vi "BeEST Temperature Logger V4 (BASVR).vi"() -> ()   [LabVIEW 2023]
uses:
  <vilib>/Utility/miscctls.llb/LVRowAndColumnTypeDef.ctl
  <vilib>/Utility/Data Type/NI_Data Type.lvlib
panel:
  out "Expected Issue":string
  in  "Tab Control":enum32{"Setup", "Run", "Advanced"}(tab)
  in  "Calibration File Path":path=path "C:/Users/CK014-user/Desktop/AVS Code V4.2/BeEST Calibration Sheet.csv"
  in  "Logging File Path":path=path "C:/Users/CK014-user/Desktop/AVS Code V4.2/BeEST Temperature Logger V4 (BASVR)/Logs/Log1.tdms"
  in  "Record Group":string="10/1/2025"
  in  "VISA RESOURCE":refnum<visa-resource-name>="COM20"
  in  "Graph Samples":T1={"Start"="0", "Max Samples"=2500000, "End"="m"} {"Max Samples" min=1}
  out "Last Y Values":i32(listbox)=3
  in  "Elapsed":bool
  in  "Graph":bool=TRUE
  in  "Record":bool=TRUE
  in  "Graph Inputs":T2={"Group"="Measured Data", "Time Track"="TIME", "Value Track"="RESISTANCE (OHMS)", "Channel Track"="CHANNEL", "Range Track"="RANGE"}
  out "Recorded\nChannels":i32(listbox)
  in  "Channel Control & Legend":i32(listbox)=2
  out "Measuring (Channel)":i32
  in  "Measure Now":u16(ring) items=["None", "0", "1", "2", "3", "4", "5", "6", "7"]
  in  "Res. to Temp.":bool=TRUE
  in  "Moving Median":u8=30 min=1
  in  "Label Precision":i32=3
  in  "Override":bool
  in  "Override Controls":T3
  in  "Generate Random AVS Data":bool
  out "Started Measuring":timestamp
  out "Resistance (Ohms)":dbl
  out "Error Code":errorcluster
  out "EXCITATION":u8
  out "Chosen Channel Index":i32
  out "XY Graph":cluster{timestamp[], "Y Array":dbl[]}[](graph)
  # "• Moving median allows you to opt for noisier, and initially more misleading, data in exchange for earlier graphing of new data if you set it especially low.\n• Graphs can fail to read if range of data is just too wide (e.g. days, at least).  This is a common, virtually inevitable bug.\n• Supposed system errors are often user errors.  Always check what calibration file you're using, what names you're using in the legend, what group you're recording, what group you're reading, etc"
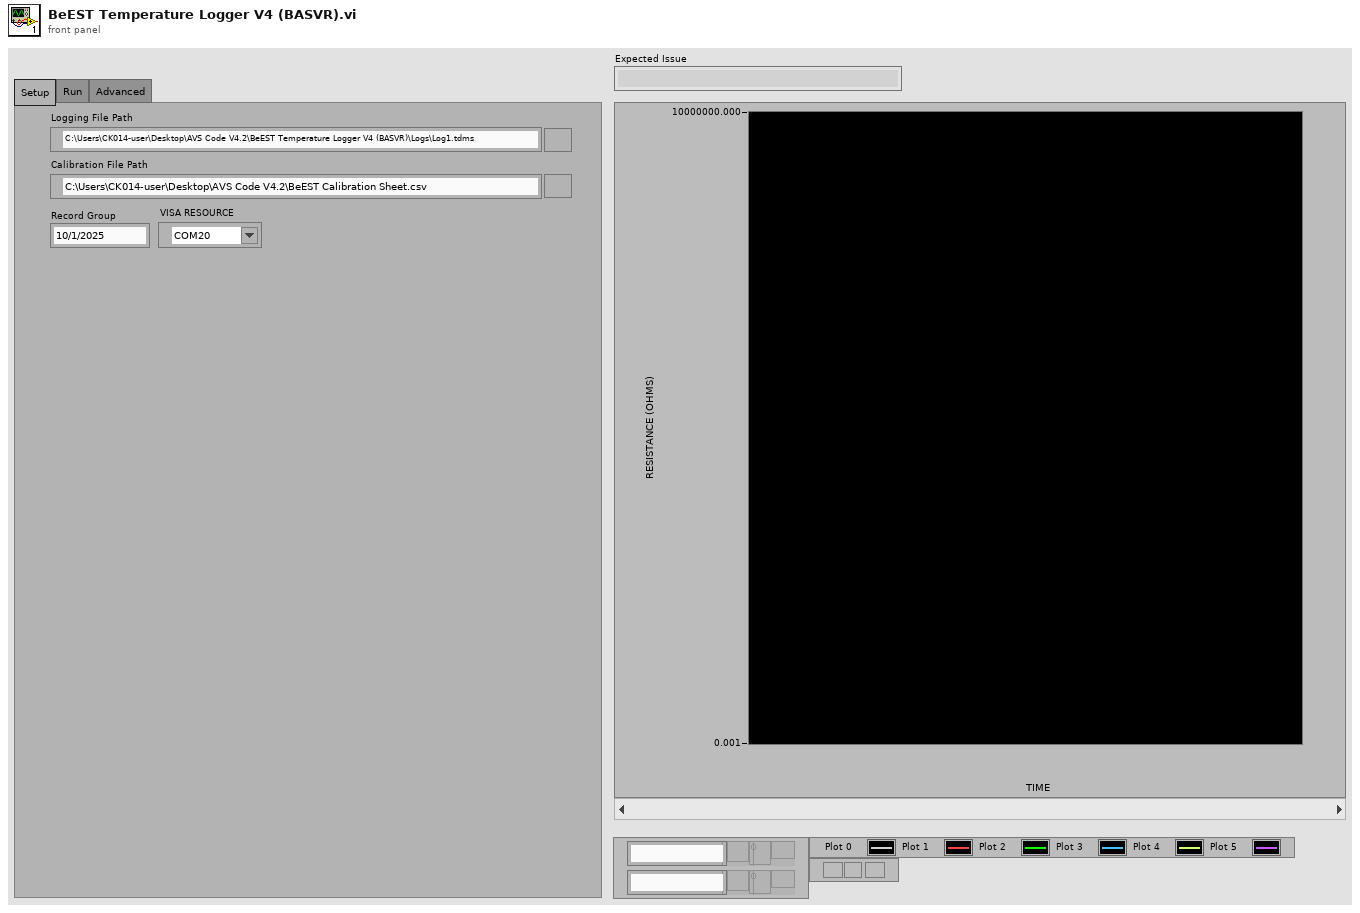
[diagram p1: front panel]
types:
  T1 = cluster{"Start":string, "Max Samples":u64, "End":string}
  T2 = cluster{"Group":string, "Time Track":string, "Value Track":string, "Channel Track":string, "Range Track":string}
  T3 = cluster{"VISA RESOURCE":refnum<visa-resource-name>, "PICOBUS ADDRESS":u8, "DISABLE AL":u8, "REMOTE":u8, "INPUT":u8, "CHANNEL":u8, "RANGE":u8, "EXCITATION":u8, "DISPLAY":u8, "DIGITAL\nREFERENCE":u16, "SET POINT":dbl, "PROP GAIN":u8, "INTG":u8, "DERIV":u8, "POWER BIAS":u8, "POWER RANGE":u8, "INFO STRING":string, "HEATER\nRESISTANCE":dbl, "INTERVAL":u8, " SENSOR dR/dT":u8}
  T4 = enum16{"open", "open or create", "create or replace", "create", "open (read-only)"}
  T5 = cluster{"Group":string, "Time Track":string, "Value Track":string, "Channel Track":string}
  T6 = cluster{"REMOTE":u8[], "RANGE":u8[], "CHANNEL":u8[], "EXCITATION":u8[], "RESISTANCE (OHMS)":sgl[], "ADC":i32[], "TIME":timestamp[]}
  T7 = cluster{"Logging File Path (last AVS loop)":path, "Logging File Refnum":refnum<k34>, "Group Name (last AVS loop)":string, "Group Name (pre-AVS-loop)":string, "Moving Median":u8, "Record":bool, "Logging File Path (current)":path, "Group Name (current)":string}
  T8 = cluster{"refnum in":refnum<k34>, "Channel Override":u16, "VISA RESOURCE":refnum<visa-resource-name>, "Channel Legend & Control":string[][], "Expected channel index":i32, "Channel Start Time":timestamp, "Measuring":i32, "Group Name":string}
  T9 = cluster{"Moving Median":u8, "Item Names":string[][], "Numeric, Timestamp, and DBL from TDML":cluster{"Integer Array":i32[], "Timestamp Array":timestamp[], "Double Array":dbl[]}, "Calibration FIle Path":path, "Elapsed?":bool, "Res. to Temp.":bool}
  T10 = typedef "LVRowAndColumnTypeDef.ctl" = cluster{"Row":i32, "Column":i32}
  T11 = cluster{"VISA RESOURCE":refnum<visa-resource-name>, "PICOBUS ADDRESS":u8, "DISABLE AL":u8, "REMOTE":u8, "INPUT":u8, "CHANNEL":u8, "RANGE":u8, "EXCITATION":u8, "DISPLAY":u8, "DIGITAL REFERENCE":u16, "SET POINT":dbl, "PROP GAIN":u8, "INTG":u8, "DERIV":u8, "POWER BIAS":u8, "POWER RANGE":u8, "INFO STRING":string, "HEATER RESISTANCE":dbl, "INTERVAL":u8, " SENSOR dR/dT":u8}
  T12 = cluster{"Integer Array":i32[], "Timestamp Array":timestamp[], "Double Array":dbl[]}
  T13 = cluster{"Channel # Column":i32[], "Valid Channel Bool 1 List":bool[], "Graph Data":cluster{timestamp[], dbl[]}[], "Internal -> Actual Channel List Index":i32[], "Internal Channel List":i32[], "Internal Channel Names":string[], "Valid Channel Bool 2 List":bool[], "Internal Channel Toggle List":string[]}
  T14 = cluster{"Name":string, "Color":u32, "Style":u8, "Point Style":u8, "Name Visible":bool, "Allow Drag":bool, "Annotation Mode":u32, "Plot":i32, "Index":i32, "Position":cluster{"X":dbl, "Y":dbl}, "X Scale":u32, "Y Scale":u32, "Show Arrow":bool, "Lock Name":bool, "Plot Area":i32, "Label Offset":cluster{"X":dbl, "Y":dbl}}[]
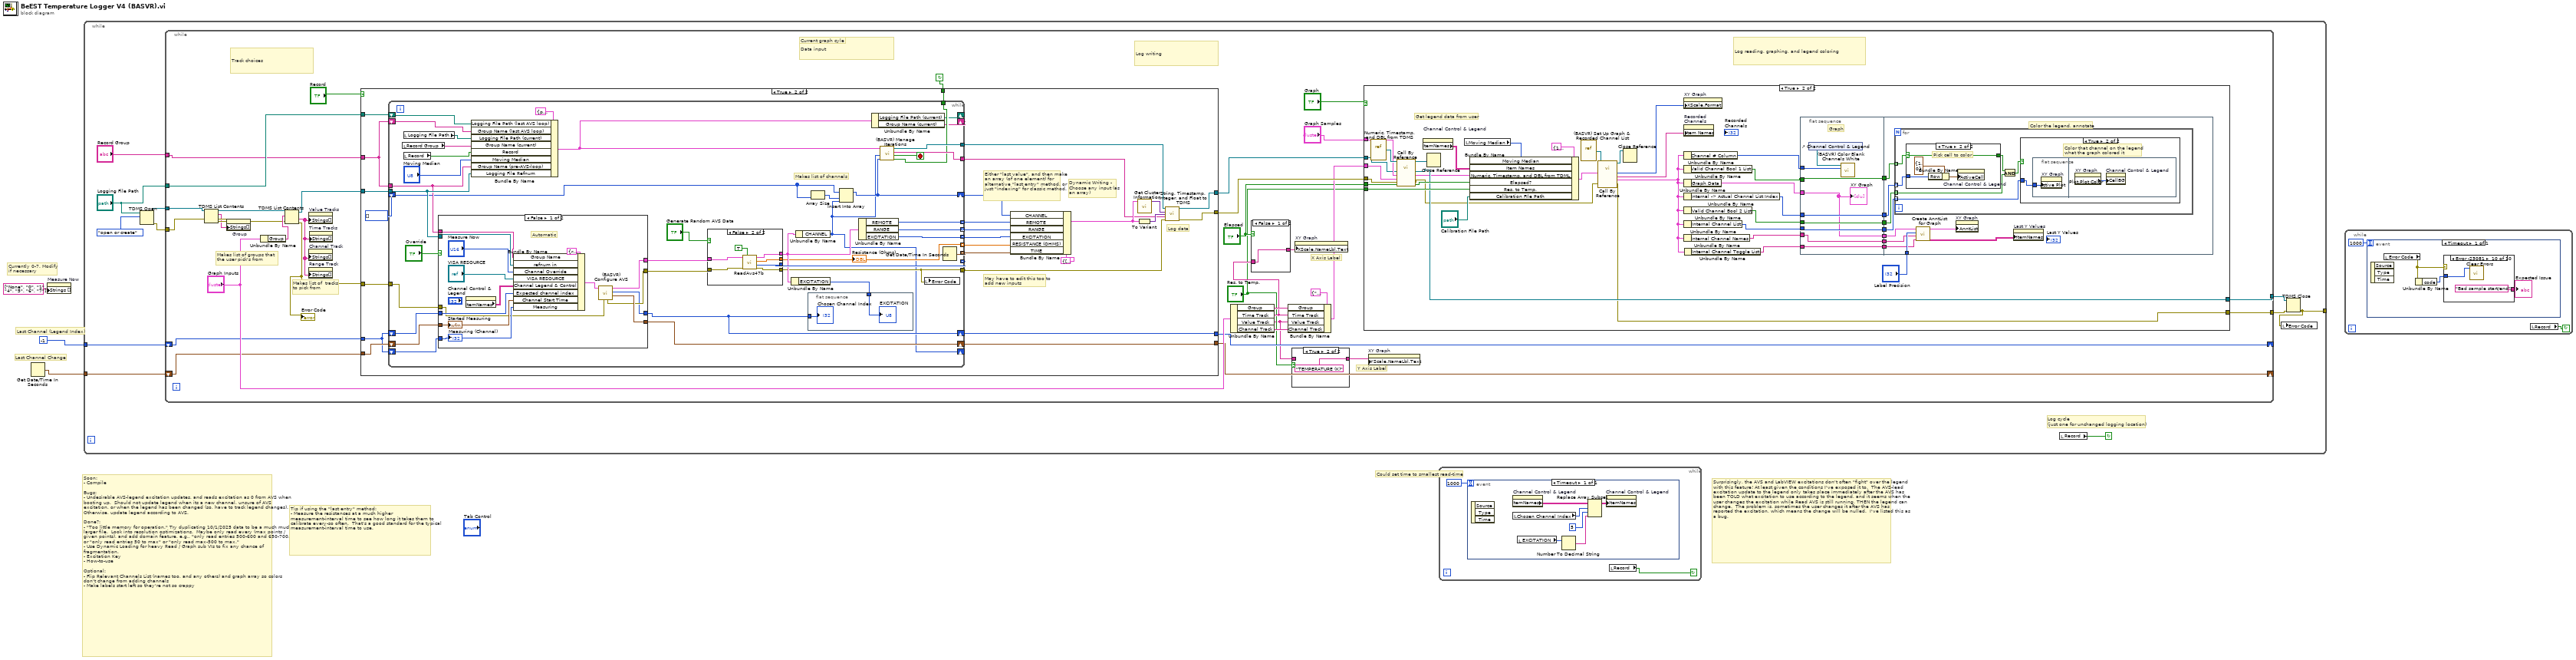
[diagram p0: block diagram]
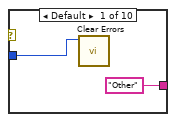
[diagram p2: hidden frame]
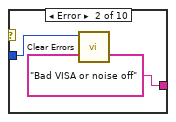
[diagram p3: hidden frame]
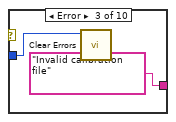
[diagram p4: hidden frame]
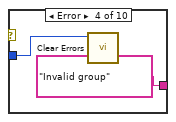
[diagram p5: hidden frame]
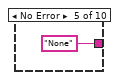
[diagram p6: hidden frame]
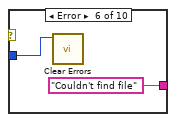
[diagram p7: hidden frame]
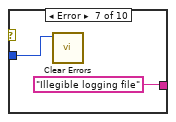
[diagram p8: hidden frame]
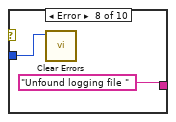
[diagram p9: hidden frame]
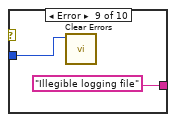
[diagram p10: hidden frame]
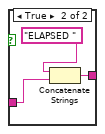
[diagram p12: hidden frame]
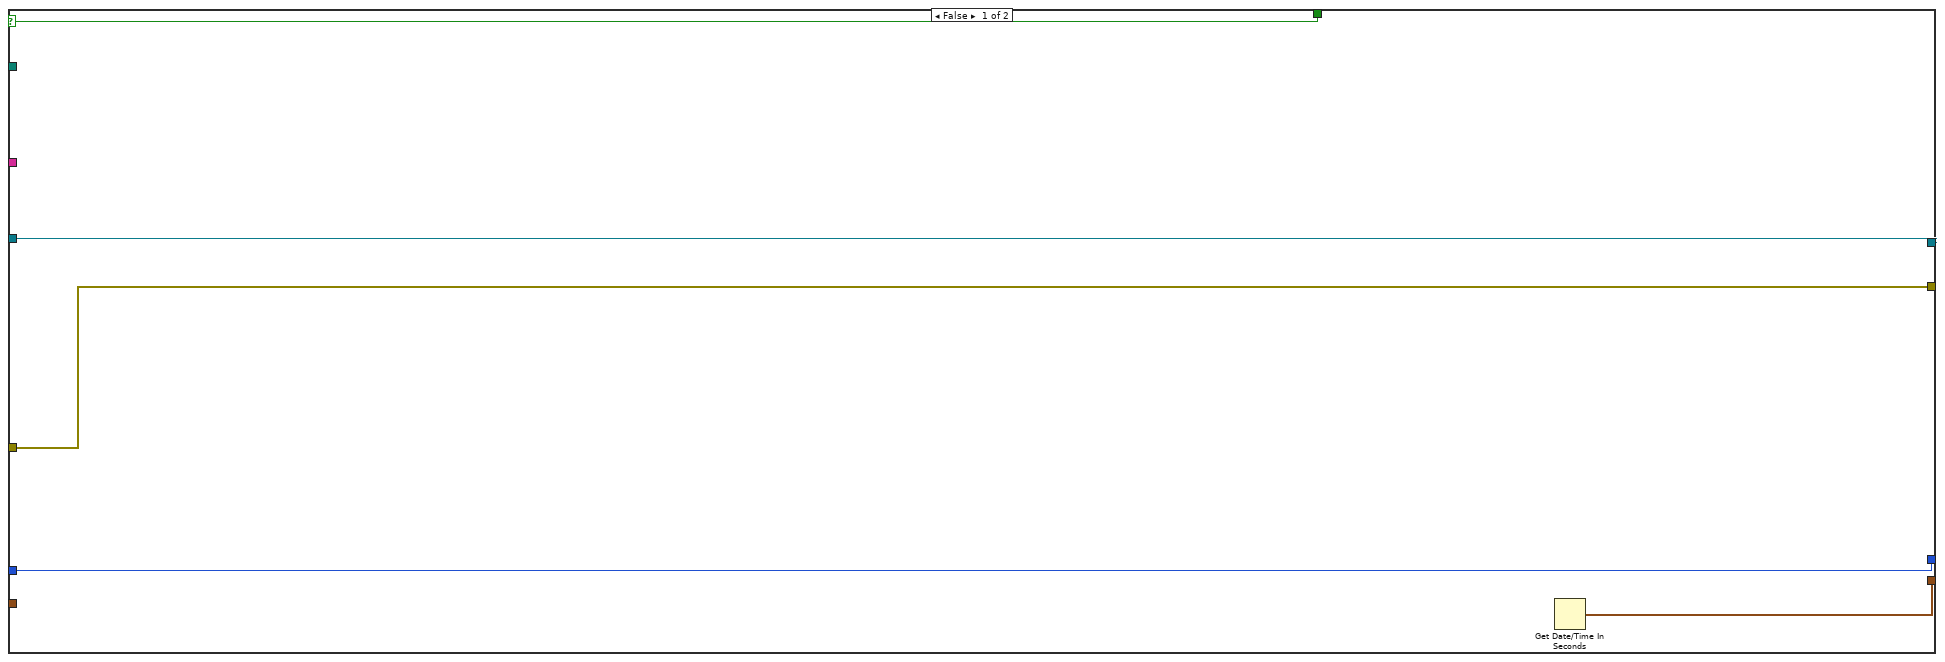
[diagram p13: hidden frame]
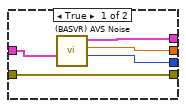
[diagram p14: hidden frame]
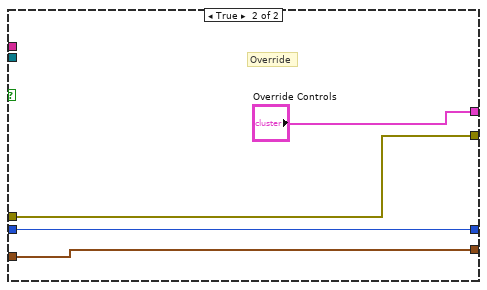
[diagram p15: hidden frame]
diagram:
  # "Surprisingly, the AVS and LabVIEW excitations don't often \"fight\" over the legend with this feature! At least given the conditions I've exposed it to.  The AVS-lead excitation update to the legend only takes place immediately after the AVS has been TOLD what excitation to use according to the legend, and it seems when the user changes the excitation while Read AVS is still running, THEN the legend can change.  The problem is, sometimes the user changes it after the AVS has reported the excitation, which means the change will be nulled.  I've listed this as a bug."
  # "Could set time to smallest read-time"
  # "Last Channel Change"
  # "Last Channel (Legend Index)"
  # "Currently 0-7. Modify if necessary"
  # "Soon: \n- Compile\n\nBugs:\n- Undesirable AVS-legend excitation updates, and reads excitation as 0 from AVS when booting up.  Should not update legend when its a new channel, unsure of AVS excitation, or when the legend has been changed (so, have to track legend changes).  Otherwise, update legend according to AVS.\n\nDone?:\n- \"Too little memory for operation.\" Try duplicating 10/1/2025 data to be a much much larger file.  Look into resolution optimizations.  Maybe only read every (max points / given points), and add domain feature, e.g., \"only read entries 500-600 and 650-700,\" or \"only read entries 50 to max\" or \"only read max-500 to max.\"\n- Use Dynamic Loading for heavy Read / Graph sub VIs to fix any chance of fragmentation.\n- Excitation Key\n- How-to-use\n\nOptional:\n- Flip Relevant Channels List (names too, and any others) and graph array so colors don't change from adding channels\n- Make labels start left so they're not so crappy"
  # "Tip if using the \"last entry\" method:\n- Measure the resistances at a much higher measurement-interval time to see how long it takes them to calibrate every-so often.  That's a good standard for the typical measurement-interval time to use."
  n1 = Get Date/Time In Seconds() -> (seconds since 1Jan1904=w3:timestamp)
  n2 = property on="Measure Now" class="Ring (strict)"("Strings []"=string[] ["None", "0", "1", "2", "3", "4", "5", "6", "7"]) -> ()  [unwired: 2 in, 2 out]
  n3 = while {
    tunnel: -1 -> [w6]
    tunnel: w3 -> [w5]
    tunnel: [w4] -> _
    stop <- w10 continue-if-true
    # "Log cycle\n(just one for unchanged logging location)"
    n4 = TDMS Open(10:T4."open or create" ("operation (0:open)"), 11:"Logging File Path") -> (0:w7:errorcluster, 3:w12:refnum<k34>)  [unwired: 5 in]
    n5 = while {
      tunnel: "Record Group" -> [w45]
      tunnel: w12 -> [w47]
      tunnel: "Logging File Path" -> [w46]
      tunnel: [w44] -> w9
      tunnel: [w43] -> w8
      tunnel: w7 -> [w42]
      shift-right: [w27] -> _
      shift-left: w6 -> [w25]
      shift-right: [w26] -> _
      shift-left: w5 -> [w24]
      stop <- w48 continue-if-true
      # "X Axis Label"
      # "Y Axis Label"
      # "Log writing"
      # "Data input"
      # "Track choices"
      # "Makes list of  tracks to pick from"
      # "Makes list of groups that the user pick's from"
      # "Log reading, graphing, and legend coloring"
      # "Current graph cyle"
      n6 = TDMS List Contents(4:w42, 7:w47) -> (0:w36:errorcluster, 2:w23:string[], 3:w38:refnum<k34>)  [unwired: 1 in, 1 out]
      n7 = property on="Group" class="CmbBox"("Strings[]"=w23) -> ()  [unwired: 2 in, 2 out]
      n8 = Unbundle By Name("Graph Inputs") -> ("Group"=w37:string)
      n9 = TDMS List Contents(4:w36, 6:w37, 7:w38) -> (0:w19:errorcluster, 1:w30:string[], 3:w35:refnum<k34>)  [unwired: 1 out]
      "Error Code" <- w19
      n10 = property on="Value Tracks" class="CmbBox"("Strings[]"=w30) -> ()  [unwired: 2 in, 2 out]
      n11 = property on="Channel Track" class="CmbBox"("Strings[]"=w30) -> ()  [unwired: 2 in, 2 out]
      n12 = property on="Range Track" class="CmbBox"("Strings[]"=w30) -> ()  [unwired: 2 in, 2 out]
      n13 = property on="Time Tracks" class="CmbBox"("Strings[]"=w30) -> ()  [unwired: 2 in, 2 out]
      n14 = case shown="True" "Record" {
        selector: "Record" -> [w57 _]
        tunnel: [w57 w71] -> w48
        tunnel: w46 -> [_ w70]
        tunnel: w45 -> [_ w69]
        tunnel: w24 -> [_ w68]
        tunnel: [w59 w67] -> w40
        tunnel: [w58 w66] -> w39
        tunnel: w35 -> [w59 w65]
        tunnel: w19 -> [w58 w64]
        tunnel: w25 -> [w56 w63]
        tunnel: [w56 w62] -> w27
        tunnel: [w55 w61] -> w26
        frame False {
          n15 = Get Date/Time In Seconds() -> (seconds since 1Jan1904=w55:timestamp)
        }
        frame True {
          # "Log data"
          # "May have to edit this too to add new inputs"
          # "Either \"last value\", and then make an array (of one element) for alternative \"last entry\" method, or just \"indexing\" for classic method."
          # "Dynamic Writing - Choose any input (as an array)"
          n16 = while {
            tunnel: [w112] -> w84 mode=indexing
            tunnel: [w123] -> _ mode=indexing
            tunnel: [w92] -> w76 mode=indexing
            tunnel: [w86] -> w81
            tunnel: [w120] -> w75 mode=indexing
            tunnel: [w110] -> w80 mode=indexing
            tunnel: [w119] -> w79 mode=indexing
            tunnel: [w104] -> w74
            tunnel: [w103] -> w73
            shift-right: [w89] -> w60
            shift-left: u8[] [] -> [w90]
            tunnel: w69 -> [w91]
            shift-right: [w100] -> _
            shift-left: w70 -> [w95]
            shift-right: [w99] -> _
            shift-left: w69 -> [w97]
            tunnel: [w101] -> w71
            shift-right: [w116] -> w61
            shift-left: w68 -> [w114]
            shift-right: [w111] -> w62
            shift-left: w63 -> [w117]
            tunnel: w65 -> [w96]
            tunnel: w64 -> [w88]
            shift-right: [w85] -> _
            shift-left: w63 -> [w115]
            stop <- w102 stop-if-true
            # "Makes list of channels"
            n17 = local read "Record Group"() -> (w107:string)
            n18 = local read "Logging File Path"() -> (w108:path)
            n19 = local read "Record"() -> (w106:bool)
            n20 = case shown="False" "Override" {
              tunnel: [w152 "Override Controls"] -> w121
              tunnel: w117 -> [w145 w154]
              tunnel: w114 -> [w144 w155]
              tunnel: [w138 w154] -> w111
              tunnel: [w151 w155] -> w116
              tunnel: w96 -> [w149 _]
              tunnel: w115 -> [w143 _]
              tunnel: w91 -> [w141 _]
              tunnel: w88 -> [w140 w153]
              tunnel: [w139 w153] -> w87
              frame False {
                # "Automatic"
                n21 = property on="Channel Control & Legend" class="MCListbox (strict)"() -> ("ItemNames"=w146:string[][])  [unwired: 2 in, 2 out]
                n22 = Bundle By Name(cluster=T8 {"refnum in"=refnum, "Channel Override"=0, "VISA RESOURCE"="COM20", "Channel Legend & Control"=[], "Expected channel index"=0, "Channel Start Time"=timestamp(0 s since 1904-01-01), "Measuring"=0, "Group Name"=""} ("input cluster"), "Group Name"=w141, "refnum in"=w149, "Channel Override"="Measure Now", "VISA RESOURCE"="VISA RESOURCE", "Channel Legend & Control"=w146, "Expected channel index"=w145, "Channel Start Time"=w144, "Measuring"=w143) -> (w142:T8)
                n23 = call "(BASVR) Configure AVS.vi"("error in (no error)"=w140, "input cluster"=w142) -> ("Channel Start Time"=w151:timestamp, "Chosen Channel Index"=w138:i32, "Configuration Cluster"=w152:T11, "error out"=w139:errorcluster)  [unwired: 5 in, 1 out]
                "Started Measuring" <- w144
                "Measuring (Channel)" <- w143
              }
              frame True {
                # "Override"
              }
            }
            n24 = Bundle By Name(cluster=T7 {"Logging File Path (last AVS loop)"=path "", "Logging File Refnum"=refnum, "Group Name (last AVS loop)"="", "Group Name (pre-AVS-loop)"="", "Moving Median"=0, "Record"=FALSE, "Logging File Path (current)"=path "", "Group Name (current)"=""}, "Logging File Path (last AVS loop)"=w95, "Group Name (last AVS loop)"=w97, "Logging File Path (current)"=w108, "Group Name (current)"=w107, "Record"=w106, "Moving Median"="Moving Median", "Group Name (pre-AVS-loop)"=w91, "Logging File Refnum"=w96) -> (w98:T7)
            n25 = case shown="False" "Generate Random AVS Data" {
              tunnel: [w130 w137] -> w93
              tunnel: [w128 w136] -> w123
              tunnel: [w126 w135] -> w86
              tunnel: w121 -> [w127 w134]
              tunnel: [w129 w133] -> w92
              tunnel: w87 -> [w126 w132]
              frame True {
                n26 = call "(BASVR) AVS Noise.vi"("AVS Input"=w127) -> ("ADC 2"=w128:i32, "Resistance"=w129:sgl, "AVS Output"=w130:T11)  [unwired: 8 in]
              }
              frame False {
                n27 = call "ReadAvs47b.vi"("SYNCHRONISE TO ADC"=TRUE, "LV ERROR IN"=w132, "CONFIGURATION CLUSTER"=w134) -> ("LV ERROR OUT"=w135:errorcluster, "ADC"=w136:i32, "RESISTANCE (OHMS)"=w133:sgl, "MODIFIED CONFIGURATION CLUSTER"=w137:T11)  [unwired: 3 in, 2 out]
              }
            }
            "Resistance (Ohms)" <- w92
            n28 = Unbundle By Name(w93) -> ("EXCITATION"=w94:u8)
            n29 = Unbundle By Name(w93) -> ("CHANNEL"=w85:u8)
            n30 = flat-sequence {
              tunnel: w94 -> [w125]
              tunnel: w111 -> [w124]
              frame #0 {
                "EXCITATION" <- w125
                "Chosen Channel Index" <- w124
              }
            }
            n31 = Array Size(array=w90) -> (size(s)=w118:i32)
            n32 = Insert Into Array(array=w90, index=w118, new element=w85) -> (w89:u8[])
            n33 = Unbundle By Name(w93) -> ("REMOTE"=w110:u8, "RANGE"=w120:u8, "EXCITATION"=w112:u8)
            n34 = Unbundle By Name(w98) -> ("Logging File Path (current)"=w100:path, "Group Name (current)"=w99:string)
            n35 = call "(BASVR) Manage Iterations.vi"("Loop's Channel List"=w89, "Current Channel"=w85, "MI Cluster"=w98) -> ("Continue current graph?"=w101:bool, "Finish AVS Loop?"=w102:bool, "group name out"=w103:string, "Logging File Refnum"=w104:refnum<k34>)  [unwired: 1 in]
            n36 = local write "Error Code"(w86) -> ()
            n37 = Get Date/Time In Seconds() -> (seconds since 1Jan1904=w119:timestamp)
          }
          n38 = Bundle By Name(cluster=T6 {"REMOTE"=[], "RANGE"=[], "CHANNEL"=[], "EXCITATION"=[], "RESISTANCE (OHMS)"=[], "ADC"=[], "TIME"=[]} ("input cluster"), "CHANNEL"=w60, "REMOTE"=w80, "RANGE"=w75, "EXCITATION"=w84, "RESISTANCE (OHMS)"=w76, "TIME"=w79) -> (w78:T6)
          n39 = call <vilib>:"Get Cluster Information.vi"("variant"=w78) -> ("cluster elements"=w83:variant[])  [unwired: 9 in, 1 out]
          n40 = To Variant(anything=w78) -> (Variant=w82:variant)
          n41 = call "String, Timestamp, Integer, and Float to TDMS.vi"("tdms file"=w74, "Data Cluster Elements"=w83, "Data Variant"=w82, "Group Name"=w73, "error in (no error)"=w81) -> ("tdms file out"=w67:refnum<k34>, "error out"=w66:errorcluster)  [unwired: 9 in]
        }
      }
      n42 = Unbundle By Name("Graph Inputs") -> ("Group"=w32:string, "Time Track"=w21:string, "Value Track"=w17:string, "Channel Track"=w34:string)
      n43 = case shown="False" "Elapsed" {
        tunnel: w21 -> [w51 w54]
        tunnel: [w51 w52] -> w20
        frame False {
        }
        frame True {
          n44 = Concatenate Strings("ELAPSED ", w54) -> (w52:string)
        }
      }
      n45 = Bundle By Name(cluster=T5 {"Group"="Measured Data", "Time Track"="", "Value Track"="", "Channel Track"=""} ("Graph Input"), "Group"=w32, "Time Track"=w21, "Value Track"=w17, "Channel Track"=w34) -> (w33:T5)
      n46 = case shown="True" "Res. to Temp." {
        tunnel: w17 -> [w49 _]
        tunnel: [w49 "TEMPERATURE (K)"] -> w16
        frame False {
        }
        frame True {
        }
      }
      n47 = property on="XY Graph" class="XYGraph (strict)"("XScale.NameLbl.Text"=w20) -> ()  [unwired: 2 in, 2 out]
      n48 = case shown="True" "Graph" {
        tunnel: w40 -> [w158 w167]
        tunnel: [w158 w172] -> w43
        tunnel: w33 -> [_ w169]
        tunnel: w39 -> [w157 w170]
        tunnel: [w157 w159] -> w44
        tunnel: "Elapsed" -> [_ w178]
        tunnel: "Res. to Temp." -> [_ w175]
        tunnel: "Graph Samples" -> [_ w168]
        frame False {
        }
        frame True {
          # "Get legend data from user"
          n49 = vi-ref "Numeric, Timestamp, and DBL from TDMS.vi"() -> (w174:refnum<vi>)
          n50 = call-by-ref "?"(reference=w174, "error in (no error)"=w170, "Group and Tracks"=w169, "Graph Samples"=w168, "Refnum in"=w167) -> (reference out=w173:refnum<vi>, "error out"=w163:errorcluster, "Numeric, Timestamp, and DBL from TDML"=w171:T12, "Refnum out"=w172:refnum<k34>)  [unwired: 6 in, 1 out]
          n51 = property on="Channel Control & Legend" class="MCListbox (strict)"() -> ("ItemNames"=w187:string[][])  [unwired: 2 in, 2 out]
          n52 = Close Reference(reference=w173) -> ()  [unwired: 1 in, 1 out]
          n53 = local read "Moving Median"() -> (w188:u8)
          n54 = Bundle By Name(cluster=T9 {"Moving Median"=15, "Item Names"=[], "Numeric, Timestamp, and DBL from TDML"={"Integer Array"=[], "Timestamp Array"=[], "Double Array"=[]}, "Calibration FIle Path"=path "", "Elapsed?"=FALSE, "Res. to Temp."=TRUE}, "Moving Median"=w188, "Item Names"=w187, "Numeric, Timestamp, and DBL from TDML"=w171, "Elapsed?"=w178, "Res. to Temp."=w175, "Calibration FIle Path"="Calibration File Path") -> (w164:T9)
          n55 = vi-ref "(BASVR) Set Up Graph & Recorded Channel List.vi"() -> (w166:refnum<vi>)
          n56 = call-by-ref "?"(reference=w166, "error In"=w163, "SUGRCL Input Cluster"=w164) -> (reference out=w165:refnum<vi>, "error out"=w159:errorcluster, "SUGRCL Output Cluster"=w160:T13, "Cleaned Channel List"=w161:string[], "X Scale.Display Format:Format"=w162:u8)  [unwired: 3 in, 1 out]
          n57 = Close Reference(reference=w165) -> ()  [unwired: 1 in, 1 out]
          n58 = property on="XY Graph" class="XYGraph (strict)"("XScale.Format"=w162) -> ()  [unwired: 2 in, 2 out]
          n59 = property on="Recorded\nChannels" class="LstBox (strict)"("Item Names"=w161) -> ()  [unwired: 2 in, 2 out]
          n60 = Unbundle By Name(w160) -> ("Channel # Column"=w179:i32[])
          n61 = Unbundle By Name(w160) -> ("Valid Channel Bool 1 List"=w180:bool[])
          n62 = Unbundle By Name(w160) -> ("Graph Data"=w181:cluster{timestamp[], dbl[]}[])
          n63 = Unbundle By Name(w160) -> ("Internal -> Actual Channel List Index"=w182:i32[])
          n64 = Unbundle By Name(w160) -> ("Valid Channel Bool 2 List"=w183:bool[])
          n65 = Unbundle By Name(w160) -> ("Internal Channel List"=w184:i32[])
          n66 = Unbundle By Name(w160) -> ("Internal Channel Names"=w185:string[])
          n67 = Unbundle By Name(w160) -> ("Internal Channel Toggle List"=w177:string[])
          n68 = flat-sequence {
            tunnel: w182 -> [w204]
            tunnel: w180 -> [w205]
            tunnel: [w205] -> w196
            tunnel: [w204] -> w195
            tunnel: w181 -> [w199]
            tunnel: w183 -> [w203]
            tunnel: [w203] -> w194
            tunnel: w184 -> [w202]
            tunnel: [w202] -> w193
            tunnel: w179 -> [w201]
            tunnel: [w199] -> w192
            tunnel: w185 -> [w198]
            tunnel: [w198] -> w191
            tunnel: w177 -> [w197]
            tunnel: [w197] -> w176
            tunnel: w196 -> [w214]
            tunnel: w195 -> [w215]
            tunnel: w194 -> [w213]
            tunnel: w193 -> [w212]
            tunnel: w192 -> [w210]
            tunnel: "Label Precision" -> [w209]
            tunnel: w191 -> [w208]
            tunnel: w176 -> [w206]
            frame #0 {
              # "Graph"
              n69 = control-ref of="Channel Control & Legend"() -> (w200:refnum<vi>)
              n70 = call "(BASVR) Color Blank Channels White.vi"("Channel # Column"=w201, "Channel Control & Legend"=w200) -> ()  [unwired: 10 in]
              "XY Graph" <- w199
            }
            frame #1 {
              # "Color the legend, annotate"
              n71 = for {
                tunnel: w213 -> [w217] mode=indexing
                tunnel: w212 -> [w221] mode=indexing
                tunnel: w215 -> [w219] mode=indexing
                tunnel: w214 -> [w218] mode=indexing
                n72 = case shown="True" w218 {
                  selector: w218 -> [w222 w224]
                  tunnel: w219 -> [_ w225]
                  tunnel: [w222 w224] -> w216
                  frame False {
                  }
                  frame True {
                    # "Pick cell to color"
                    n73 = Bundle By Name(cluster=T10 {"Row"=1, "Column"=0} ("Active Cell:Active Cell"), "Row"=w225) -> (w223:T10)
                    n74 = property on="Channel Control & Legend" class="MCListbox (strict)"("ActiveCell"=w223) -> ()  [unwired: 2 in, 2 out]
                  }
                }
                n75 = And(x=w216, y=w217) -> (x .and. y?=w220:bool)
                n76 = case shown="True" w220 {
                  tunnel: w221 -> [_ w227]
                  frame False {
                  }
                  frame True {
                    # "Color that channel on the legend what the graph colored it"
                    n77 = flat-sequence {
                      tunnel: w227 -> [w228]
                      frame #0 {
                        n78 = property on="XY Graph" class="XYGraph (strict)"("Active Plot"=w228) -> ()  [unwired: 2 in, 2 out]
                      }
                      frame #1 {
                        n79 = property on="XY Graph" class="XYGraph (strict)"() -> ("Plot.Plot Color"=w229:u32)  [unwired: 2 in, 2 out]
                        n80 = property on="Channel Control & Legend" class="MCListbox (strict)"("CellBG"=w229) -> ()  [unwired: 2 in, 2 out]
                      }
                    }
                  }
                }
              }
              n81 = call "Create AnntList for Graph.vi"("Internal Channel Toggle List"=w206, "Internal Channel Name List"=w208, "Label Precision"=w209, "Graph Input"=w210) -> ("Last Measurements"=w207:string[][], "AnntList Input"=w211:T14)  [unwired: 6 in]
              n82 = property on="XY Graph" class="XYGraph (strict)"("AnntList"=w211) -> ()  [unwired: 2 in, 2 out]
              n83 = property on="Last Y Values" class="MCListbox (strict)"("ItemNames"=w207) -> ()  [unwired: 2 in, 2 out]
            }
          }
        }
      }
      n84 = property on="XY Graph" class="XYGraph (strict)"("YScale.NameLbl.Text"=w16) -> ()  [unwired: 2 in, 2 out]
    }
    n85 = local read "Record"() -> (w10:bool)
    n86 = TDMS Close(8:w9, 11:w8) -> (0:w4:errorcluster)  [unwired: 1 out]
    n87 = local write "Error Code"(w4) -> ()
  }
  n88 = while {
    stop <- w230 continue-if-true
    n89 = event shown="[0] Timeout" {
      selector: _ -> [_]
      dyn-events: _ -> [_]
      timeout: 1000 -> [_]
      event Timeout {
        n90 = event-data() -> ()  [unwired: 1 in, 3 out]
        n91 = property on="Channel Control & Legend" class="MCListbox (strict)"() -> ("ItemNames"=w237:string[][])  [unwired: 2 in, 2 out]
        n92 = local read "Chosen Channel Index"() -> (w236:i32)
        n93 = local read "EXCITATION"() -> (w234:u8)
        n94 = Number To Decimal String(number=w234) -> (decimal integer string=w233:string)  [unwired: 1 in]
        n95 = Replace Array Subset(array=w237, new element=w233, index (row)=w236, index (col)=5 ("disabled index (col)")) -> (w232:string[][])
        n96 = property on="Channel Control & Legend" class="MCListbox (strict)"("ItemNames"=w232) -> ()  [unwired: 2 in, 2 out]
      }
    }
    n97 = local read "Record"() -> (w230:bool)
  }
  n98 = while {
    stop <- w239 continue-if-true
    n99 = event shown="[0] Timeout" {
      selector: _ -> [_]
      dyn-events: _ -> [_]
      timeout: 1000 -> [_]
      event Timeout {
        n100 = event-data() -> ()  [unwired: 1 in, 3 out]
        n101 = local read "Error Code"() -> (w241:errorcluster)
        n102 = Unbundle By Name(w241) -> ("code"=w240:i32)
        n103 = case shown="Error -23081" w241 {
          tunnel: ["Other" "Bad VISA or noise off" "Invalid calibration file" "Invalid group" "None" ("Message") "Couldn't find file" ("Message") "Illegible logging file" ("Message") "Unfound logging file " ("Message") "Illegible logging file" "Bad sample start/end"] -> w242
          tunnel: w240 -> [w243 w245 w248 w250 _ w252 w255 w257 w258 w261]
          frame Default {
            n104 = call <vilib>:"Clear Errors.vi"("specific error code to clear (0: all)"=w243) -> ()  [unwired: 5 in, 2 out]
          }
          frame Error {
            n105 = call <vilib>:"Clear Errors.vi"("specific error code to clear (0: all)"=w245) -> ()  [unwired: 5 in, 2 out]
          }
          frame Error {
            n106 = call <vilib>:"Clear Errors.vi"("specific error code to clear (0: all)"=w248) -> ()  [unwired: 5 in, 2 out]
          }
          frame Error {
            n107 = call <vilib>:"Clear Errors.vi"("specific error code to clear (0: all)"=w250) -> ()  [unwired: 5 in, 2 out]
          }
          frame No Error {
          }
          frame Error {
            n108 = call <vilib>:"Clear Errors.vi"("specific error code to clear (0: all)"=w252) -> ()  [unwired: 5 in, 2 out]
          }
          frame Error {
            n109 = call <vilib>:"Clear Errors.vi"("specific error code to clear (0: all)"=w255) -> ()  [unwired: 5 in, 2 out]
          }
          frame Error {
            n110 = call <vilib>:"Clear Errors.vi"("specific error code to clear (0: all)"=w257) -> ()  [unwired: 5 in, 2 out]
          }
          frame Error {
            n111 = call <vilib>:"Clear Errors.vi"("specific error code to clear (0: all)"=w258) -> ()  [unwired: 5 in, 2 out]
          }
          frame Error {
            n112 = call <vilib>:"Clear Errors.vi"("specific error code to clear (0: all)"=w261) -> ()  [unwired: 5 in, 2 out]
          }
        }
        "Expected Issue" <- w242
      }
    }
    n113 = local read "Record"() -> (w239:bool)
  }
